vi "findSystemFolder.vi"(5 "error in (no error)":errorcluster, 6 "system directory type":T1 items=["User Home"=0, "User Desktop"=1, "User Documents"=2, "User Application Data"=3, "User Preferences"=4, "User Temporary"=5, "Public Documents"=6, "Public Application Data"=7, "Public Preferences"=8, "Public Cache"=13, "System Core Libraries"=9, "System Installed Libraries"=10, "Application Files"=11, "Boot Volume Root"=12], 7 "Application Name":string="Unknown") -> (13 "App Folder":path, 19 "error out":errorcluster)   [LabVIEW 2022 SP3, in "stillnessHelper.lvclass"]
uses:
  stillnessHelper.lvclass
  <vilib>/Utility/sysdir.llb/System Directory Type.ctl
  <userlib>/_OpenG.lib/file/file.llb/File Exists - Scalar__ogtk.vi
  <userlib>/_OpenG.lib/file/file.llb/openg_file.lvlib
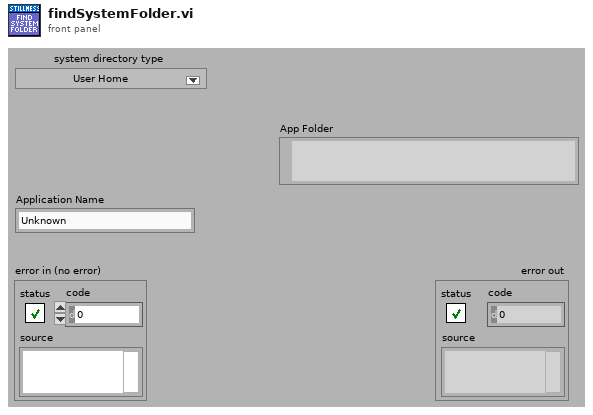
[diagram p1: front panel]
types:
  T1 = typedef "System Directory Type.ctl" = i32
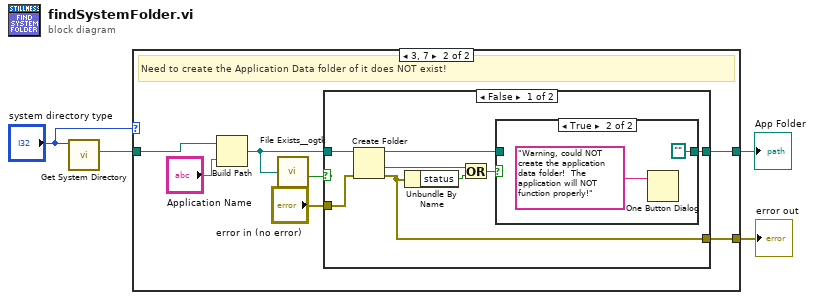
[diagram p0: block diagram]
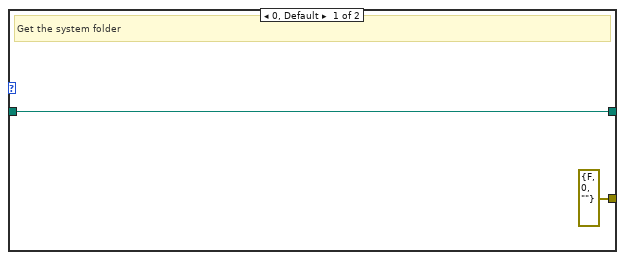
[diagram p2: hidden frame]
diagram:
  n1 = call <vilib>:"Get System Directory.vi"("system directory type"="system directory type") -> ("system directory"=w3:path)  [unwired: 10 in]
  n2 = case shown="3, 7" "system directory type" {
    tunnel: [errorcluster {"status"=FALSE, "code"=0, "source"=""} ("error in (no error)") w13] -> w4
    tunnel: w3 -> [w6 w11]
    tunnel: [w6 w10] -> w2
    frame 0, Default {
      # "Get the system folder"
    }
    frame 3, 7 {
      # "Need to create the Application Data folder of it does NOT exist!"
      n3 = Build Path(base path=w11, name or relative path="Application Name") -> (appended path=w7:path)
      n4 = call-poly <userlib>:"File Exists__ogtk.vi"("file path"=w7) -> ("exists"=w8:bool)  [unwired: 6 in, 1 out]
      n5 = case shown="False" w8 {
        tunnel: w7 -> [w21 w26]
        tunnel: [w17 w26] -> w10
        tunnel: "error in (no error)" -> [w15 w25]
        tunnel: [w14 w25] -> w13
        frame False {
          n6 = Create Folder(path (use dialog)=w21, error in=w15) -> (created path=w16:path, cancelled=w20:bool, error out=w14:errorcluster)  [unwired: 1 in]
          n7 = Unbundle By Name(w14) -> ("status"=w19:bool)
          n8 = Or(x=w20, y=w19) -> (x .or. y?=w18:bool)
          n9 = case shown="True" w18 {
            tunnel: [w22 path ""] -> w17
            tunnel: w16 -> [w22 _]
            frame False {
            }
            frame True {
              n10 = One Button Dialog(message="Warning, could NOT create the application data folder!  The application will NOT function properly!") -> ()  [unwired: 1 in, 1 out]
            }
          }
        }
        frame True {
        }
      }
    }
  }
  "App Folder" <- w2
  "error out" <- w4
